vi "Time.Timestamps to Duration, HHMMSS.vi"(9 "Start":timestamp, 11 "End":timestamp) -> (0 "Secs":dbl, 1 "Mins":dbl, 2 "Hours":dbl, 3 "Duration":string, 5 "Total Secs":dbl format="%#.3f")   [LabVIEW 2024, in "EQMF.lvlib" / "Time Utils.lvlib"]
uses:
  Time Utils.lvlib
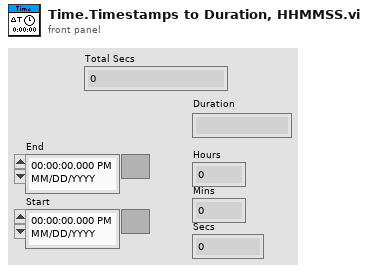
[diagram p1: front panel]
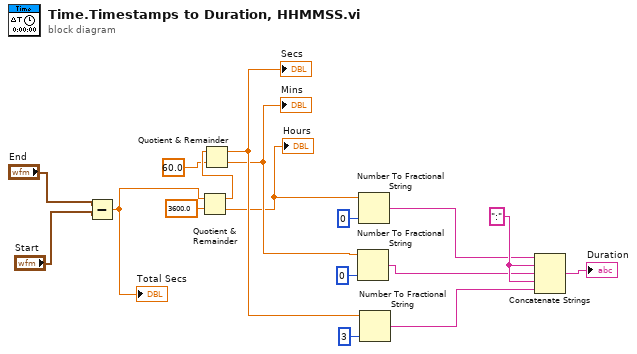
[diagram p0: block diagram]
diagram:
  w4 = ":"
  n1 = Subtract(x="End", y="Start") -> (x-y=w12:dbl)
  "Total Secs" <- w12
  n2 = Quotient & Remainder(x=w12, y=3600.0) -> (x-y*floor(x/y)=w16:dbl, floor(x/y)=w6:dbl)
  "Hours" <- w6
  n3 = Quotient & Remainder(x=w16, y=60.0) -> (x-y*floor(x/y)=w11:dbl, floor(x/y)=w7:dbl)
  "Mins" <- w7
  "Secs" <- w11
  n4 = Number To Fractional String(number=w7, precision (6)=i16 0) -> (F-format string=w2:string)  [unwired: 2 in]
  n5 = Number To Fractional String(number=w6, precision (6)=i16 0) -> (F-format string=w3:string)  [unwired: 2 in]
  n6 = Number To Fractional String(number=w11, precision (6)=i16 3) -> (F-format string=w1:string)  [unwired: 2 in]
  n7 = Concatenate Strings(w3, w4, w2, w4, w1) -> (→"Duration":string)
